vi "Post-Build Action.vi"(5 "Files Generated by Build":path[](array[path]), 6 "Top Level/Always Included VIs":path[](array[path]), 7 "Destination Path":path, 8 "error in (no error)":errorcluster, 9 "Target Name":string, 10 "Build Specification Name":string, 11 "Project Path":path) -> (0 "error out":errorcluster)   [LabVIEW 2022 SP3]
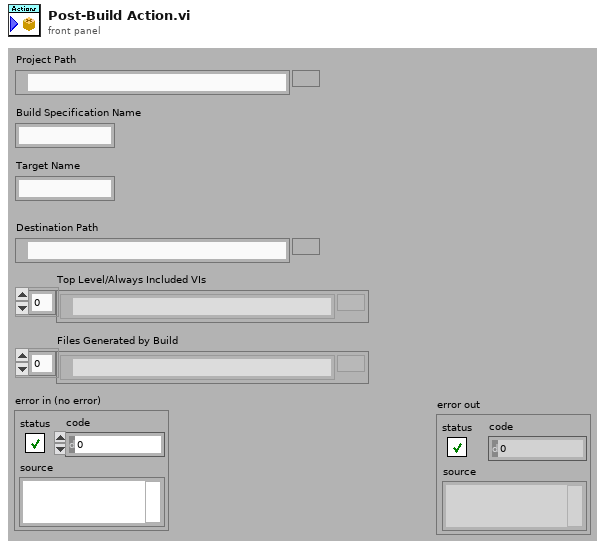
[diagram p1: front panel]
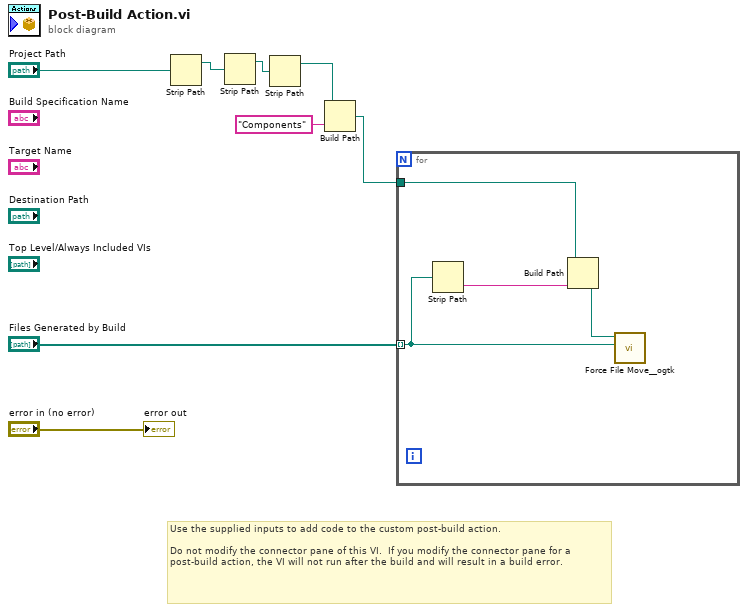
[diagram p0: block diagram]
diagram:
  # "Use the supplied inputs to add code to the custom post-build action.\n\nDo not modify the connector pane of this VI.  If you modify the connector pane for a post-build action, the VI will not run after the build and will result in a build error."
  n1 = Strip Path(path="Project Path") -> (stripped path=w5:path)  [unwired: 1 out]
  n2 = Strip Path(path=w5) -> (stripped path=w4:path)  [unwired: 1 out]
  n3 = Strip Path(path=w4) -> (stripped path=w3:path)  [unwired: 1 out]
  n4 = Build Path(base path=w3, name or relative path="Components") -> (appended path=w6:path)
  n5 = for {
    tunnel: "Files Generated by Build" -> [w11] mode=indexing
    tunnel: w6 -> [w12]
    n6 = Strip Path(path=w11) -> (name=w10:string)  [unwired: 1 out]
    n7 = Build Path(base path=w12, name or relative path=w10) -> (appended path=w9:path)
    n8 = call <userlib>:"Force File Move__ogtk.vi"("source"=w11, "target"=w9) -> ()  [unwired: 4 in, 2 out]
  }
  "error out" <- "error in (no error)"
